vi "Global_An_Out_Var.vi"() -> ()   [LabVIEW 2016, in "DNP3_Master_Station_Template.lvlib"]
uses:
  <vilib>/DNP3/DNP3_Master/Analog Variation.ctl
  DNP3_Master_Station_Template.lvlib
  <vilib>/DNP3/DNP3_Master.lvlib
panel:
  in  "Analog Out Variation":T1=4 items=["32-bit"=1, "16-bit"=2, "Single-prec"=3, "Double-prec"=4]
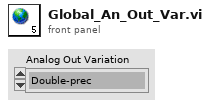
[diagram p1: front panel]
types:
  T1 = typedef "DNP3_Master.lvlib/Analog Variation.ctl" = u8
diagram:
